vi "Initialize Default.vi"(8 "error in":errorcluster, 11 "RDMA Tx Transfer Configuration in":refnum<class "RDMA Transfer Tx Configuration.lvclass">) -> (0 "error out":errorcluster, 3 "RDMA Tx Transfer Configuration out":refnum<class "RDMA Transfer Tx Configuration.lvclass">)   [LabVIEW 2020, in "RDMA.lvlib" / "RDMA Transfer Tx Configuration.lvclass"]
uses:
  RDMA Transfer Tx Configuration.lvclass
  Tx Transfer Settings.ctl
  RDMA Transfer Tx Configuration.lvclass/RDMA Transfer Tx Configuration.ctl
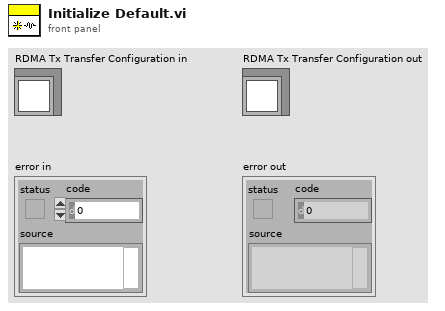
[diagram p1: front panel]
types:
  T1 = typedef "RDMA.lvlib/RDMA Transfer Tx Configuration.lvclass/Tx Transfer Settings.ctl" = cluster{"local address":u32, "local port":u16, "destination address":u32, "destination port":u16}
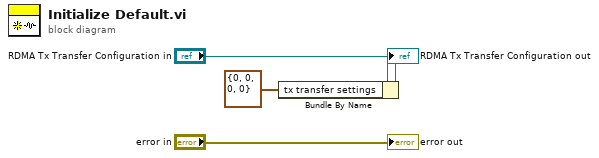
[diagram p0: block diagram]
diagram:
  n1 = Bundle By Name(cluster="RDMA Tx Transfer Configuration in", "tx transfer settings"=T1 {"local address"=0, "local port"=0, "destination address"=0, "destination port"=0}) -> (→"RDMA Tx Transfer Configuration out":refnum<class "RDMA Transfer Tx Configuration.lvclass">)
  "error out" <- "error in"
